vi "Move Asset.vi"(8 "error in (no error)":errorcluster, 10 "Serial Number":string="1234", 11 "Part Number":string="B0CG1KL3RC") -> (0 "error out":errorcluster, 3 "asset id":string="2d7e2a0f-e140-47e2-ae68-ae9bd23d949b")   [LabVIEW 2024]
panel:
  in  "Physical Location":string
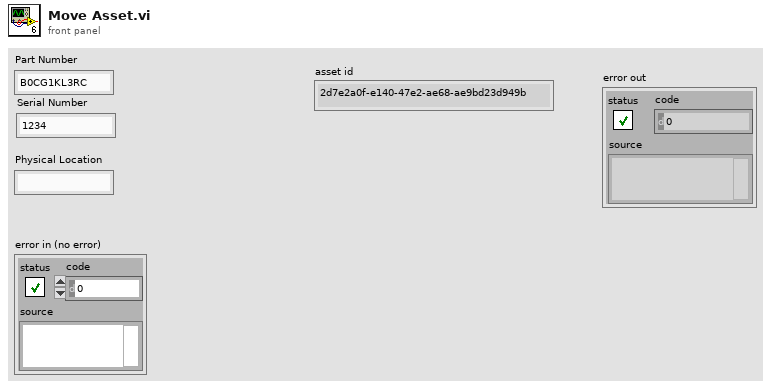
[diagram p1: front panel]
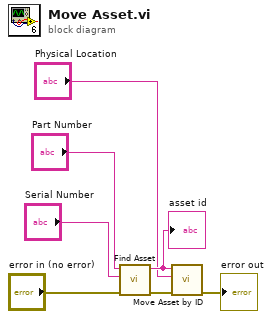
[diagram p0: block diagram]
diagram:
  n1 = call "Find Asset.vi"("error in (no error)"="error in (no error)", "Serial Number"="Serial Number", "Part Number"="Part Number") -> ("error out"=w3:errorcluster, "Asset ID"=w4:string)  [unwired: 6 in, 1 out]
  "asset id" <- w4
  n2 = call "Move Asset by ID.vi"("error in (no error)"=w3, "Physical Location"="Physical Location", "Asset ID"=w4) -> ("error out"=→"error out":errorcluster)  [unwired: 8 in]
